vi "Dual AIN Loop.vi"() -> (0 "error out":errorcluster)   [LabVIEW 2009]
panel:
  out "Elapsed Time Text":string="0  00:00:05"
  out "Elapsed Time Text":string="0  00:00:19"
  in  "stop 2":bool
  out "Waveform Chart":cluster{"Value Read":dbl, "Value Read":dbl}(graph)={"Value Read"=-0.019768353551626205, "Value Read"=-0.01872771792113781}
  in  "stop":bool
  in  "Interval [ms]":i32
  in  "# Channels":i32=6
  in  "Channel Names":string[](array[string])=["AIN0", "AIN1", "AIN2", "AIN3", "AIN4", "AIN5"]
  in  "Config Values":dbl[](array[numeric])=[199.0, 10.0, 0.0, 199.0, 10.0, 0.0] format="%.2f"
  out "Error String":string="No Error"
  out "ConnectionType Out":i32=4
  out "DeviceType Out":i32=7
  in  "Identifier":string="192.168.0.101"
  in  "ConnectionType":string="Wifi"
  in  "DeviceType":string="T7"
  in  "Config NumFrames":i32=6
  out "Values":dbl[](array[numeric])=[-0.019768353551626205, -0.01872771792113781] format="%.6f"
  in  "Config Names":string[](array[string])=["AIN0_NEGATIVE_CH", "AIN0_RANGE", "AIN0_RESOLUTION_INDEX", "AIN1_NEGATIVE_CH", "AIN1_RANGE", "AIN1_RESOLUTION_INDEX"]
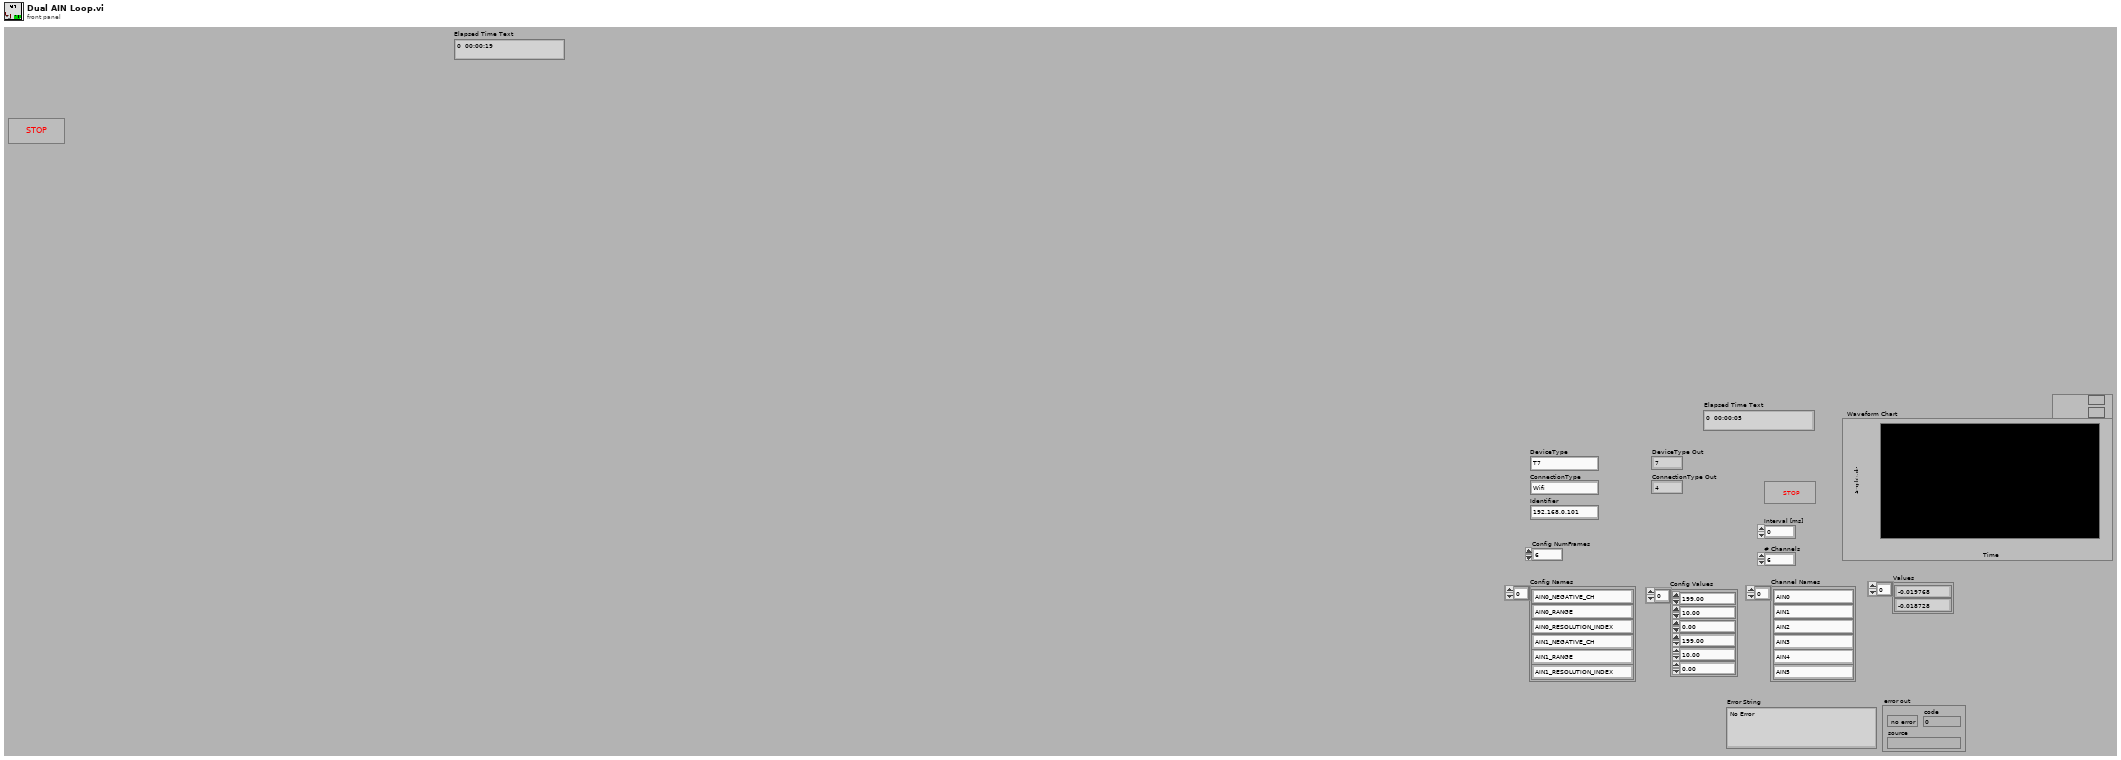
[diagram p1: front panel]
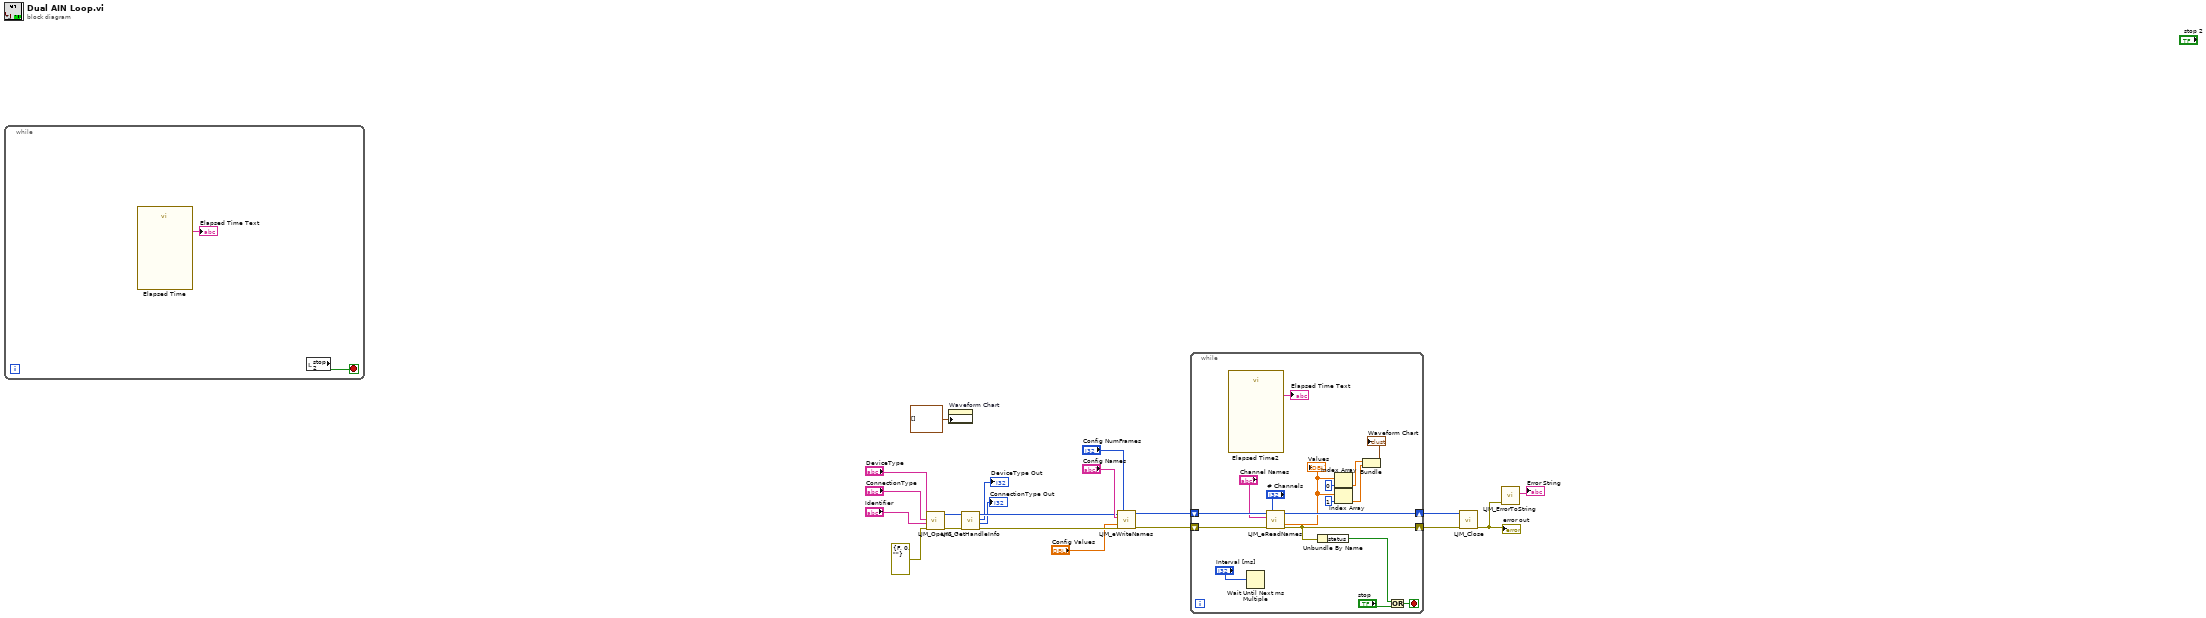
[diagram p0: block diagram]
diagram:
  n1 = while {
    stop <- w22 stop-if-true
    n2 = call "Elapsed Time"() -> ("Elapsed Time Text"=→"Elapsed Time Text":string)  [unwired: 12 in, 7 out]
    n3 = local read "stop 2"() -> (w22:bool)
  }
  n4 = call <vilib>:"LJM_OpenS.vi"("error in"=errorcluster {"status"=FALSE, "code"=0, "source"=""} ("error in (no error)"), "Identifier"="Identifier", "ConnectionType"="ConnectionType", "DeviceType"="DeviceType") -> ("error out"=w17:errorcluster, "Handle"=w15:i32)  [unwired: 6 in]
  n5 = property on="Waveform Chart" class="WaveformChart (strict)"("History Data"=cluster{"Value Read":dbl, "Value Read":dbl}[] []) -> ()  [unwired: 2 in, 2 out]
  n6 = call <vilib>:"LJM_GetHandleInfo.vi"("error in"=w17, "Handle In"=w15) -> ("error out"=w16:errorcluster, "ConnectionType"=→"ConnectionType Out":i32, "DeviceType"=→"DeviceType Out":i32, "Handle Out"=w14:i32)  [unwired: 2 in, 4 out]
  n7 = call <vilib>:"LJM_eWriteNames.vi"("Handle In"=w14, "NumFrames"="Config NumFrames", "aNames"="Config Names", "aValuesIn"="Config Values", "error in"=w16) -> ("Handle Out"=w4:i32, "error out"=w5:errorcluster)  [unwired: 8 in, 1 out]
  n8 = while {
    shift-left: w4 -> [w38]
    shift-right: [w37] -> w2
    shift-left: w5 -> [w39]
    shift-right: [w31] -> w3
    stop <- w33 stop-if-true
    n9 = call "Elapsed Time2"() -> ("Elapsed Time Text"=→"Elapsed Time Text":string)  [unwired: 12 in, 7 out]
    n10 = Wait Until Next ms Multiple(millisecond multiple="Interval [ms]") -> ()  [unwired: 1 out]
    n11 = call <vilib>:"LJM_eReadNames.vi"("Handle In"=w38, "NumFrames"="# Channels", "aNames"="Channel Names", "error in"=w39) -> ("Handle Out"=w37:i32, "aValuesOut"=w25:dbl[], "error out"=w31:errorcluster)  [unwired: 8 in, 1 out]
    "Values" <- w25
    n12 = Unbundle By Name(w31) -> ("status"=w32:bool)
    n13 = Index Array(array=w25, index=0 ("Index")) -> (element=w27:dbl)
    n14 = Index Array(array=w25, index=1 ("Index")) -> (element=w26:dbl)
    n15 = Bundle("Numeric"=w27, "Numeric"=w26) -> (→"Waveform Chart":cluster{"Numeric":dbl, "Numeric":dbl})  [unwired: 1 in]
    n16 = Or(x=w32, y="stop") -> (x .or. y?=w33:bool)
  }
  n17 = call <vilib>:"LJM_Close.vi"("error in"=w3, "Handle"=w2) -> ("error out"=w8:errorcluster)  [unwired: 9 in]
  "error out" <- w8
  n18 = call <vilib>:"LJM_ErrorToString.vi"("error in"=w8) -> ("String"=→"Error String":string)  [unwired: 10 in]
